vi "ADPcms.vi"() -> ()   [LabVIEW 2019]
uses:
  <vilib>/Instr/_visa.llb/VISA Configure Serial Port (Instr).vi
  <vilib>/Utility/file.llb/Write Delimited Spreadsheet (string).vi
  <vilib>/Utility/file.llb/Write Delimited Spreadsheet (DBL).vi
panel:
  out "Lux Chart":dbl(graph)
  out "Humidity Chart":dbl(graph)
  out "Water Alarm":bool
  out "Lux Alarm":bool
  out "UV Alarm":bool
  out "Temp Alarm":bool
  out "Humid Alarm":bool
  out "Water Warning":bool
  out "Lux Warning":bool
  out "UV Warning":bool
  out "Temp Warning":bool
  out "Humid Warning":bool
  out "Data: Time, Humidity, Temperature, UV, Lux, Water Level":dbl[][](array[numeric])
  in  "Water Level Standard":dbl
  out "Water Level Accuracy (%)":dbl
  out "Water Level":dbl
  in  "Calibrate Water Level Characterization":bool
  out "Water Level":dbl
  out "Lux Value":dbl
  out "UV Value":dbl
  out "Temperature (F)":dbl
  out "Humidity":dbl
  out "Current Time":dbl
  in  "Temperature Standard":dbl
  out "Temperature Accuracy (%)":dbl
  in  "Diagnostics Mode":bool
  out "Temperature (F)":dbl
  in  "Calibrate Temperature Bias":bool
  out "Arduino Power":bool
  in  "Calibration Mode":bool
  in  "Operational Mode":bool
  out "Elapsed Time (s)":dbl
  in  "?":bool
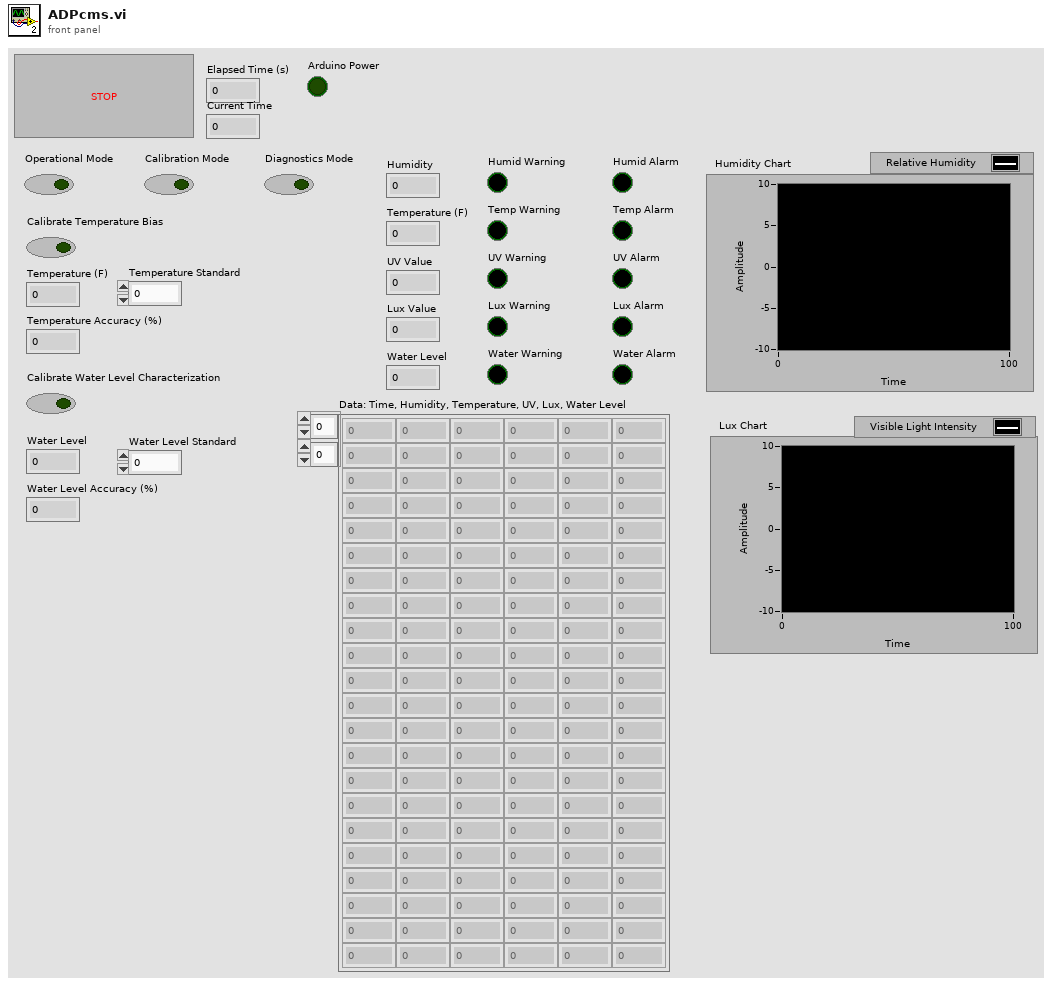
[diagram p1: front panel]
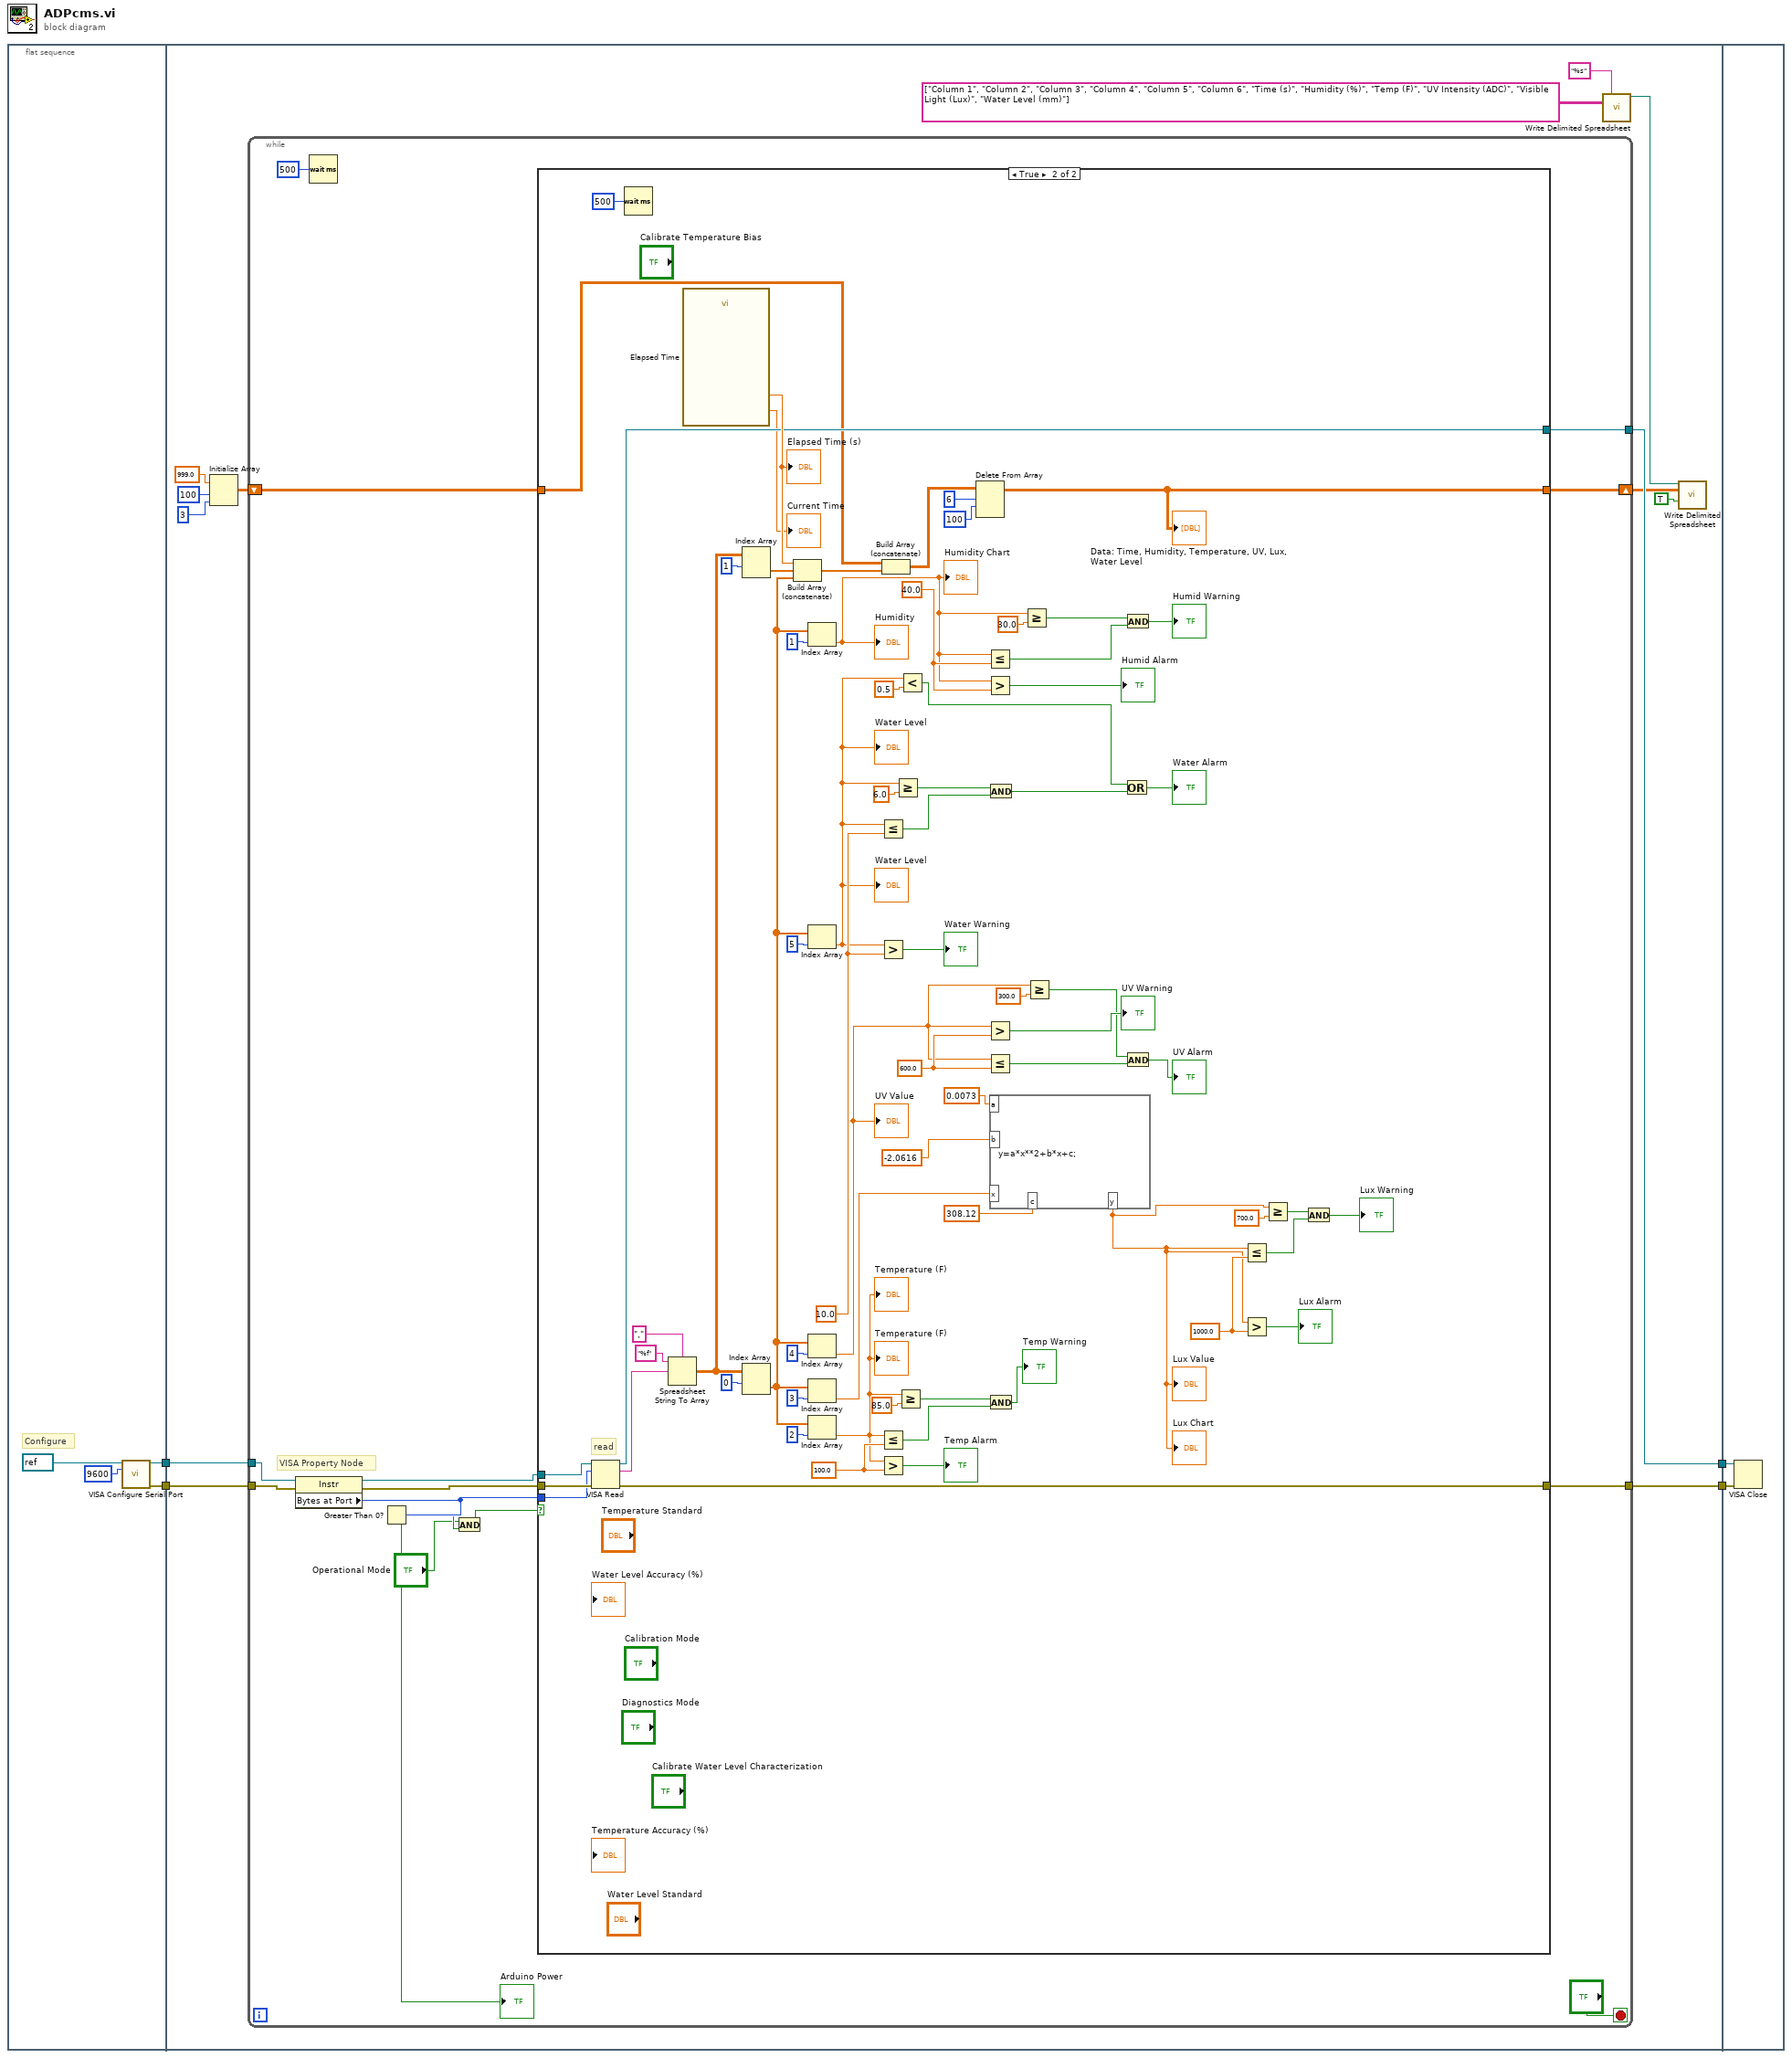
[diagram p0: block diagram]
diagram:
  n1 = flat-sequence {
    tunnel: [w6] -> w4
    tunnel: [w5] -> w3
    tunnel: w4 -> [w18]
    tunnel: w3 -> [w17]
    tunnel: [w16] -> w2
    tunnel: [w15] -> w1
    tunnel: w2 -> [w108]
    tunnel: w1 -> [w109]
    frame #0 {
      # "Configure"
      n2 = call-poly "VISA Configure Serial Port"("VISA resource name"=refnum<visa-resource-name> refnum, "baud rate (9600)"=u32 9600) -> ("VISA resource name out"=w6:refnum<visa-resource-name>, "error out"=w5:errorcluster)  [unwired: 12 in]
    }
    frame #1 {
      n3 = Initialize Array(999.0 ("element"), 100 ("dimension size"), 3 ("dimension size")) -> (w14:dbl[][])
      n4 = while {
        tunnel: w18 -> [w35]
        tunnel: w17 -> [w34]
        tunnel: [w32] -> w16
        tunnel: [w30] -> w15
        shift-right: [w22] -> w9
        shift-left: w14 -> [w23]
        stop <- "?" stop-if-true
        # "VISA Property Node"
        n5 = property class="Instr"(reference=w35, error in=w34) -> (reference out=w31:refnum<visa-resource-name>, error out=w29:errorcluster, "Bytes at Port"=w28:u32)
        n6 = Wait (ms)(milliseconds to wait=u32 500) -> ()  [unwired: 1 out]
        n7 = Greater Than 0?(x=w28) -> (x > 0?=w27:bool)
        "Arduino Power" <- w27
        n8 = And(x="Operational Mode", y=w27) -> (x .and. y?=w25:bool)
        n9 = case shown="True" w25 {
          tunnel: [w38 w89] -> w32
          tunnel: w31 -> [w38 w99]
          tunnel: [w37 w88] -> w30
          tunnel: w29 -> [w37 w98]
          tunnel: w28 -> [_ w97]
          tunnel: w23 -> [w36 w86]
          tunnel: [w36 w64] -> w22
          frame False {
          }
          frame True {
            w43 = 10.0 ("y")
            w50 = 100.0 ("y")
            w57 = 600.0 ("y")
            w70 = 1000.0 ("y")
            w81 = 40.0 ("y")
            # "read"
            n10 = VISA Read(VISA resource name=w99, byte count=w97, error in (no error)=w98) -> (VISA resource name out=w89:refnum<visa-resource-name>, read buffer=w107:string, error out=w88:errorcluster)  [unwired: 1 out]
            n11 = Wait (ms)(milliseconds to wait=u32 500) -> ()  [unwired: 1 out]
            n12 = Spreadsheet String To Array(delimiter (Tab)=",", format string="%f", spreadsheet string=w107) -> (array=w101:dbl[][])  [unwired: 1 in]
            n13 = call "Elapsed Time"() -> ("Present (s)"=→"Current Time":dbl, "Elapsed Time (s)"=w90:dbl)  [unwired: 12 in, 6 out]
            "Elapsed Time (s)" <- w90
            n14 = Index Array(array=w101, index (row)=1) -> (element=w102:dbl[])  [unwired: 1 in]
            n15 = Index Array(array=w101, index (row)=0) -> (element=w95:dbl[])  [unwired: 1 in]
            n16 = Build Array (concatenate)(w90, w102, w95) -> (w87:dbl[])
            n17 = Index Array(array=w95, index=1) -> (element=w79:dbl)
            "Humidity" <- w79
            "Humidity Chart" <- w79
            n18 = Index Array(array=w95, index=5) -> (element=w39:dbl)
            "Water Level" <- w39
            "Water Level" <- w39
            n19 = Index Array(array=w95, index=4) -> (element=w56:dbl)
            "UV Value" <- w56
            n20 = Index Array(array=w95, index=3) -> (element=w78:dbl)
            n21 = Index Array(array=w95, index=2) -> (element=w49:dbl)
            "Temperature (F)" <- w49
            "Temperature (F)" <- w49
            n22 = Less Or Equal?(x=w39, y=w43) -> (x <= y?=w41:bool)
            n23 = Greater?(x=w39, y=w43) -> (0:→"Water Warning":bool)
            n24 = Less Or Equal?(x=w49, y=w50) -> (x <= y?=w54:bool)
            n25 = Greater?(x=w49, y=w50) -> (0:→"Temp Alarm":bool)
            n26 = Build Array (concatenate)(w86, w87) -> (w65:dbl[][])
            n27 = Greater Or Equal?(x=w39, y=6.0) -> (x >= y?=w40:bool)
            n28 = Greater Or Equal?(x=w49, y=85.0) -> (x >= y?=w53:bool)
            n29 = Less?(x=w39, y=0.5) -> (x < y?=w47:bool)
            n30 = Delete From Array(array=w65, length=6, index (row)=100) -> (array with subset deleted=w64:dbl[][])  [unwired: 1 in, 1 out]
            "Data: Time, Humidity, Temperature, UV, Lux, Water Level" <- w64
            n31 = Less Or Equal?(x=w79, y=w81) -> (x <= y?=w84:bool)
            n32 = Greater?(x=w79, y=w81) -> (0:→"Humid Alarm":bool)
            n33 = Greater?(x=w56, y=w57) -> (0:→"UV Warning":bool)
            n34 = Less Or Equal?(x=w56, y=w57) -> (x <= y?=w59:bool)
            n35 = And(x=w40, y=w41) -> (x .and. y?=w46:bool)
            n36 = And(x=w53, y=w54) -> (x .and. y?=→"Temp Warning":bool)
            n37 = formula code="y=a*x**2+b*x+c;"("a"=0.0073 ("input variable"), "x"=w78, "b"=-2.0616 ("input variable"), "c"=308.12 ("input variable")) -> ("y"=w69:dbl)
            "Lux Value" <- w69
            "Lux Chart" <- w69
            n38 = Greater Or Equal?(x=w79, y=30.0) -> (x >= y?=w85:bool)
            n39 = Greater Or Equal?(x=w56, y=300.0) -> (x >= y?=w58:bool)
            n40 = Or(x=w47, y=w46) -> (x .or. y?=→"Water Alarm":bool)
            n41 = And(x=w85, y=w84) -> (x .and. y?=→"Humid Warning":bool)
            n42 = And(x=w58, y=w59) -> (x .and. y?=→"UV Alarm":bool)
            n43 = Less Or Equal?(x=w69, y=w70) -> (x <= y?=w73:bool)
            n44 = Greater?(x=w69, y=w70) -> (0:→"Lux Alarm":bool)
            n45 = Greater Or Equal?(x=w69, y=700.0) -> (x >= y?=w72:bool)
            n46 = And(x=w72, y=w73) -> (x .and. y?=→"Lux Warning":bool)
          }
        }
      }
      n47 = call-poly <vilib>:"Write Delimited Spreadsheet.vi"("format (%s)"="%s", "2D data"=string[][] [["Column 1", "Column 2", "Column 3", "Column 4", "Column 5", "Column 6"], ["Time (s)", "Humidity (%)", "Temp (F)", "UV Intensity (ADC)", "Visible Light (Lux)", "Water Level (mm)"]]) -> ("new file path (Not A Path if cancelled)"=w11:path)  [unwired: 12 in, 1 out]
      n48 = call-poly <vilib>:"Write Delimited Spreadsheet.vi"("file path (dialog if empty)"=w11, "2D data"=w9, "append to file? (new file:F)"=TRUE) -> ()  [unwired: 11 in, 2 out]
    }
    frame #2 {
      n49 = VISA Close(VISA resource name=w108, error in (no error)=w109) -> ()  [unwired: 1 out]
    }
  }
